vi "test-SwerveDrvPoseEst2-Test2.vi"(8 "error in (no error)":errorcluster) -> (0 "error out":errorcluster, 3 "Test Passed":bool)   [LabVIEW 2019]
uses:
  <vilib>/Rock Robotics/WPI/ThirdParty/JAS_Junk/TrajLib/Trajectory_Library.lvlib
panel:
  out "max x error":dbl
  out "max y err":dbl
  out "Y Error":dbl[](array[numeric])
  out "X error":dbl[](array[numeric])
  out "Total":i32
  out "Total passed":i32
  out "Sub error":bool
  out "End Y pos passed":bool
  out "End X pos passed":bool
  out "AddVisionCount":i32
  out "TotalTImeSecs 2":dbl
  out "BenchProcessing \nTimer Per Pass":dbl
  out "BenchTotalTime":dbl
  out "BenchTotalPasses":dbl
  out "MaxErrPassed":bool
  out "MeanPassed":bool
  out "ErrorSumNormalized":dbl
  out "Error Sum":dbl
  out "Max Error":dbl
  out "VIsionMeasCount":i32
  out "TotalTImeSecs":dbl
  out "Position Graph":cluster{dbl[], dbl[]}[](graph)
  out "PoseEst2NewErr":errorcluster
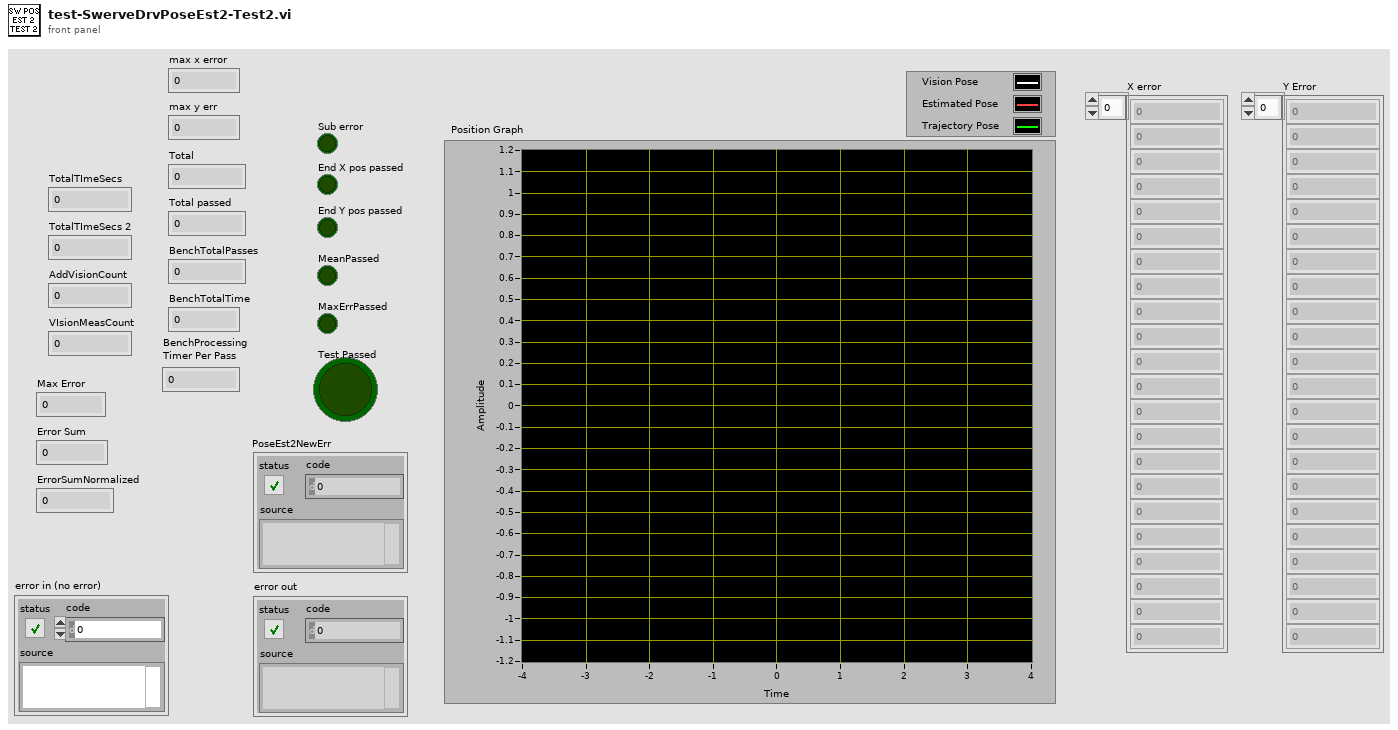
[diagram p1: front panel]
types:
  T1 = typedef "Trajectory_Library.lvlib/TRANSLATION2D.ctl" = cluster{"X":dbl, "Y":dbl}
  T2 = typedef "Trajectory_Library.lvlib/ROTATION2D.ctl" = cluster{"VALUE":dbl, "COS":dbl, "SIN":dbl}
  T3 = typedef "Trajectory_Library.lvlib/SWERVE_DRIVE_MODULE_POSITION.ctl" = cluster{"Distance":dbl, "Angle":T2, "P":bool}
  T4 = typedef "Trajectory_Library.lvlib/SWERVE_DRIVE_KINEMATICS.ctl" = cluster{"NumModules":i32, "InverseKinematics":T5, "ForwardKinematics":T5, "Modules":T1[], "PrevCoR":T1, "SavedModuleStates":T6[]}
  T5 = typedef "NI_Matrix.lvlib/RealMatrix.ctl" = dbl[][]
  T6 = typedef "Trajectory_Library.lvlib/SWERVE_DRIVE_MODULE_STATE.ctl" = cluster{"Speed":dbl, "Angle":T2}
  T7 = typedef "Trajectory_Library.lvlib/POSE2D.ctl" = cluster{"TRANSLATION":T1, "ROTATION":T2}
  T8 = typedef "Trajectory_Library.lvlib/TRAJ_CONFIG.ctl" = cluster{"MaxVelocity":dbl, "Max Acceleration":dbl, "StartVelocity":dbl, "End Velocity":dbl, "Reversed":bool, "Constraints":variant[]}
  T9 = typedef "Trajectory_Library.lvlib/SWERVE_DRIVE_POSE_EST2.ctl" = cluster{"M_Vision_K":T5, "m_nominal_dT":dbl, "m_PrevTime_Sec":dbl, "Pose_Buffer":T10, "Swerve_Drive_Kinematics":T4, "Swerve_Drive_Odom":T11, "M_Q":T5, "NumModules":i32}
  T10 = typedef "Trajectory_Library.lvlib/TIME_INTERPOLATABLE_VARIANT.ctl" = cluster{"TimeStamps":dbl[], "DataArray":variant[], "Min_TimeStamp":dbl, "Max_TimeStamp":dbl, "ItemCount":i32, "MaxBufferTime":dbl}
  T11 = typedef "Trajectory_Library.lvlib/SWERVE_DRIVE_ODOMETRY.ctl" = cluster{"POSE":T7, "GyroOffset":T2, "PreviousAngle":T2, "PrevModulePositions":T3[], "NumModules":i32}
  T12 = typedef "Trajectory_Library.lvlib/TRAJECTORY.ctl" = cluster{"TotalTImeSecs":dbl, "States":T13[]}
  T13 = typedef "Trajectory_Library.lvlib/TRAJ_STATE.ctl" = cluster{"TimeSeconds":dbl, "Velocity":dbl, "Acceleration":dbl, "POSE":T7, "Curvature":dbl}
  T14 = typedef "Trajectory_Library.lvlib/TRANSFORM2D.ctl" = cluster{"TRANSLATION":T1, "ROTATION":T2, "xF":bool}
  T15 = cluster{"MaxErrPassed":bool, "MeanPassed":bool, "Error Sum":dbl, "ErrorSumNormalized":dbl, "Max Error":dbl, "AddVisionCount":i32, "VIsionApplyCount":i32, "BenchTotalPasses":dbl, "BenchTotalTime":dbl, "BenchProcessing \nTimer Per Pass":dbl, "TotalTImeSecs":dbl, "End X pos passed":bool, "End Y pos passed":bool, "Sub error":bool, "End X Dev":dbl, "End Y Dev":dbl}
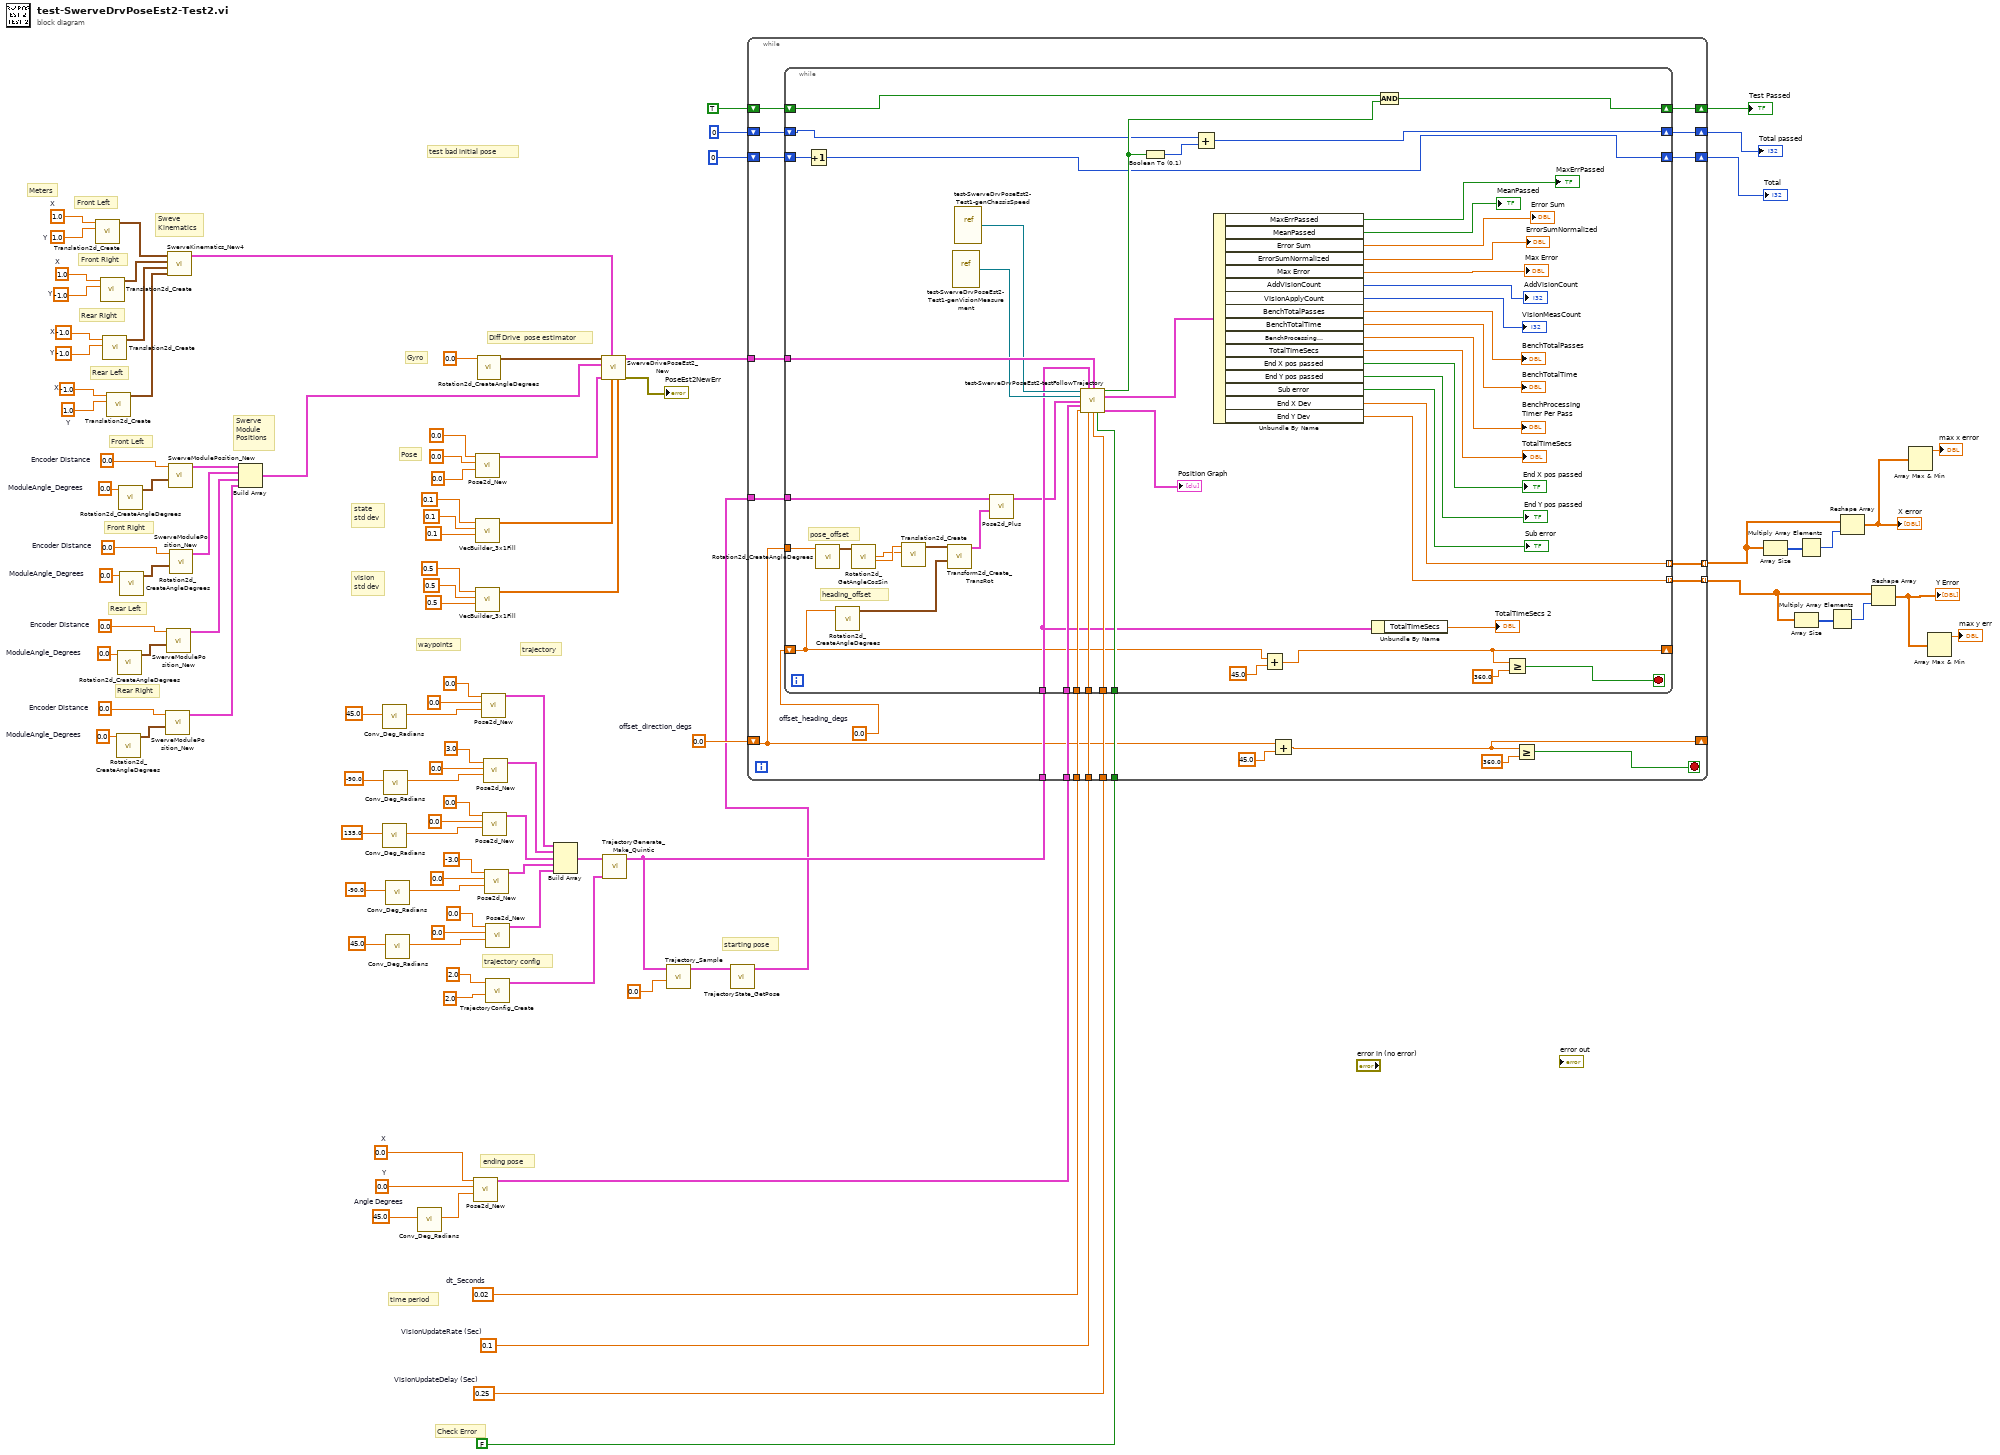
[diagram p0: block diagram]
diagram:
  w10 = -1.0  # X
  w9 = 1.0  # Y
  w8 = -1.0  # X
  w7 = -1.0  # Y
  w6 = 1.0  # X
  w5 = -1.0  # Y
  w4 = 1.0  # X
  w3 = 1.0  # Y
  w27 = 0.0  # ModuleAngle_Degrees
  w25 = 0.0  # Encoder Distance
  w24 = 0.0  # ModuleAngle_Degrees
  w22 = 0.0  # Encoder Distance
  w21 = 0.0  # ModuleAngle_Degrees
  w19 = 0.0  # Encoder Distance
  w17 = 0.0  # ModuleAngle_Degrees
  w15 = 0.0  # Encoder Distance
  w48 = 0.0  # offset_direction_degs
  w53 = 0.25  # VisionUpdateDelay (Sec)
  w54 = 0.1  # VisionUpdateRate (Sec)
  w59 = 0.0  # X
  w58 = 0.0  # Y
  w56 = 45.0  # Angle Degrees
  w60 = 0.02  # dt_Seconds
  # "Meters"
  # "Sweve\nKinematics"
  # "Rear Right"
  # "Rear Left"
  # "Front Right"
  # "Front Left"
  # "Front Left"
  # "Swerve\nModule\nPositions"
  # "Rear Right"
  # "Rear Left"
  # "Front Right"
  # "test bad initial pose"
  # "starting pose"
  # "Check Error"
  # "ending pose"
  # "state \nstd dev"
  # "time period"
  # "vision \nstd dev"
  # "Pose"
  # "Gyro"
  # "Diff Drive  pose estimator"
  # "trajectory config"
  # "trajectory"
  # "waypoints"
  n1 = call <vilib>:"Translation2d_Create.vi"("Y"=w3, "X"=w4) -> ("TRANSLATION"=w11:T1)  [unwired: 9 in]
  n2 = call <vilib>:"Translation2d_Create.vi"("Y"=w5, "X"=w6) -> ("TRANSLATION"=w12:T1)  [unwired: 9 in]
  n3 = call <vilib>:"Translation2d_Create.vi"("Y"=w7, "X"=w8) -> ("TRANSLATION"=w13:T1)  [unwired: 9 in]
  n4 = call <vilib>:"Translation2d_Create.vi"("Y"=w9, "X"=w10) -> ("TRANSLATION"=w14:T1)  [unwired: 9 in]
  n5 = call <vilib>:"Rotation2d_CreateAngleDegrees.vi"("Angle_Degrees"=w27) -> ("ROTATION"=w26:T2)  [unwired: 10 in]
  n6 = call <vilib>:"Rotation2d_CreateAngleDegrees.vi"("Angle_Degrees"=w24) -> ("ROTATION"=w23:T2)  [unwired: 10 in]
  n7 = call <vilib>:"Rotation2d_CreateAngleDegrees.vi"("Angle_Degrees"=w17) -> ("ROTATION"=w16:T2)  [unwired: 10 in]
  n8 = call <vilib>:"Rotation2d_CreateAngleDegrees.vi"("Angle_Degrees"=w21) -> ("ROTATION"=w20:T2)  [unwired: 10 in]
  n9 = call <vilib>:"SwerveModulePosition_New.vi"("ROTATION"=w26, "Distance"=w25) -> ("SWERVE_DRIVE_MODULE_POSITION"=w30:T3)  [unwired: 9 in]
  n10 = call <vilib>:"SwerveModulePosition_New.vi"("ROTATION"=w23, "Distance"=w22) -> ("SWERVE_DRIVE_MODULE_POSITION"=w29:T3)  [unwired: 9 in]
  n11 = call <vilib>:"SwerveKinematics_New4.vi"("wheel 3"=w14, "wheel 2"=w13, "wheel 1"=w12, "wheel 0"=w11) -> ("SWERVE_DRIVE_KINEMATICS"=w2:T4)  [unwired: 7 in]
  n12 = call <vilib>:"SwerveModulePosition_New.vi"("ROTATION"=w16, "Distance"=w15) -> ("SWERVE_DRIVE_MODULE_POSITION"=w18:T3)  [unwired: 9 in]
  n13 = call <vilib>:"SwerveModulePosition_New.vi"("ROTATION"=w20, "Distance"=w19) -> ("SWERVE_DRIVE_MODULE_POSITION"=w28:T3)  [unwired: 9 in]
  n14 = Build Array(w18, w28, w29, w30) -> (w1:T3[])
  n15 = call <vilib>:"Conv_Deg_Radians.vi"("Degress"=45.0 ("Heading")) -> ("Radians"=w82:dbl)  [unwired: 10 in]
  n16 = call <vilib>:"Conv_Deg_Radians.vi"("Degress"=135.0 ("Heading")) -> ("Radians"=w90:dbl)  [unwired: 10 in]
  n17 = call <vilib>:"Conv_Deg_Radians.vi"("Degress"=-90.0 ("Heading")) -> ("Radians"=w86:dbl)  [unwired: 10 in]
  n18 = call <vilib>:"Conv_Deg_Radians.vi"("Degress"=-90.0 ("Heading")) -> ("Radians"=w94:dbl)  [unwired: 10 in]
  n19 = call <vilib>:"Conv_Deg_Radians.vi"("Degress"=45.0 ("Heading")) -> ("Radians"=w98:dbl)  [unwired: 10 in]
  n20 = call <vilib>:"Conv_Deg_Radians.vi"("Degress"=w56) -> ("Radians"=w57:dbl)  [unwired: 10 in]
  n21 = call <vilib>:"Pose2d_New.vi"("Heading"=w57, "Y"=w58, "X"=w59) -> ("out POSe"=w55:T7)  [unwired: 8 in]
  n22 = call <vilib>:"Pose2d_New.vi"("Heading"=0.0, "Y"=0.0, "X"=0.0) -> ("out POSe"=w68:T7)  [unwired: 8 in]
  n23 = call <vilib>:"VecBuilder_3x1Fill.vi"("R2"=0.1 ("element"), "R1"=0.1 ("element"), "R0"=0.1 ("element")) -> ("output matrix"=w63:T5)  [unwired: 8 in]
  n24 = call <vilib>:"VecBuilder_3x1Fill.vi"("R2"=0.5 ("element"), "R1"=0.5 ("element"), "R0"=0.5 ("element")) -> ("output matrix"=w62:T5)  [unwired: 8 in]
  n25 = call <vilib>:"Rotation2d_CreateAngleDegrees.vi"("Angle_Degrees"=0.0) -> ("ROTATION"=w67:T2)  [unwired: 10 in]
  n26 = call <vilib>:"Pose2d_New.vi"("Heading"=w82, "Y"=0.0, "X"=0.0) -> ("out POSe"=w81:T7)  [unwired: 8 in]
  n27 = call <vilib>:"Pose2d_New.vi"("Heading"=w90, "Y"=0.0, "X"=0.0) -> ("out POSe"=w78:T7)  [unwired: 8 in]
  n28 = call <vilib>:"Pose2d_New.vi"("Heading"=w86, "Y"=0.0, "X"=3.0) -> ("out POSe"=w79:T7)  [unwired: 8 in]
  n29 = call <vilib>:"Pose2d_New.vi"("Heading"=w94, "Y"=0.0, "X"=-3.0) -> ("out POSe"=w77:T7)  [unwired: 8 in]
  n30 = call <vilib>:"Pose2d_New.vi"("Heading"=w98, "Y"=0.0, "X"=0.0) -> ("out POSe"=w103:T7)  [unwired: 8 in]
  n31 = call <vilib>:"TrajectoryConfig_Create.vi"("MaxAcceleration"=2.0, "MaxVelocity"=2.0) -> ("TRAJECTORY_CONFIG"=w100:T8)  [unwired: 9 in]
  n32 = Build Array(w81, w79, w78, w77, w103) -> (w101:T7[])
  n33 = call <vilib>:"SwerveDrivePoseEst2_New.vi"("VisionMeasurementStdDevs"=w62, "StateStdDevs"=w63, "SWERVE_DRIVE_KINEMATICS"=w2, "InitialPose"=w68, "Module Positions"=w1, "gyroAngle"=w67) -> ("Error"=→"PoseEst2NewErr":errorcluster, "SwerveDrivePoseEstimate"=w61:T9)  [unwired: 4 in]
  n34 = call <vilib>:"TrajectoryGenerate_Make_Quintic.vi"("traj_config"=w100, "waypointPOSE"=w101) -> ("TRAJECTORY"=w51:T12)  [unwired: 8 in, 1 out]
  n35 = call <vilib>:"Trajectory_Sample.vi"("Time"=0.0, "InputTRAJECTORY"=w51) -> ("OutputTRAJ_STATE"=w49:T13)  [unwired: 9 in]
  n36 = call <vilib>:"TrajectoryState_GetPose.vi"("TRAJ_STATE"=w49) -> ("TrajStatePose"=w47:T7)  [unwired: 10 in]
  n37 = while {
    tunnel: w61 -> [w127]
    tunnel: w60 -> [w126]
    tunnel: w55 -> [w125]
    tunnel: w54 -> [w124]
    tunnel: w53 -> [w123]
    tunnel: FALSE -> [w122]
    tunnel: w51 -> [w121]
    shift-right: [w116] -> _
    shift-left: w48 -> [w114]
    tunnel: w47 -> [w115]
    shift-right: [w112] -> w45
    shift-left: TRUE -> [w113]
    shift-right: [w110] -> w43
    shift-left: 0 -> [w111]
    shift-right: [w108] -> w41
    shift-left: 0 -> [w109]
    tunnel: [w107] -> w39 mode=indexing
    tunnel: [w106] -> w35 mode=indexing
    stop <- w118 stop-if-true
    w117 = 0.0  # offset_heading_degs
    n38 = while {
      tunnel: w127 -> [w177]
      tunnel: w126 -> [w176]
      tunnel: w125 -> [w175]
      tunnel: w124 -> [w174]
      tunnel: w123 -> [w173]
      tunnel: w122 -> [w171]
      tunnel: w121 -> [w153]
      shift-right: [w148] -> _
      shift-left: w117 -> [w146]
      tunnel: w115 -> [w139]
      tunnel: w114 -> [w144]
      shift-right: [w136] -> w112
      shift-left: w113 -> [w137]
      shift-right: [w132] -> w110
      shift-left: w111 -> [w134]
      shift-right: [w130] -> w108
      shift-left: w109 -> [w131]
      tunnel: [w129] -> w107 mode=indexing
      tunnel: [w128] -> w106 mode=indexing
      stop <- w149 stop-if-true
      # "heading_offset"
      # "pose_offset"
      n39 = Increment(x=w131) -> (x+1=w130:i32)
      n40 = call <vilib>:"Rotation2d_CreateAngleDegrees.vi"("Angle_Degrees"=w144) -> ("ROTATION"=w145:T2)  [unwired: 10 in]
      n41 = call <vilib>:"Rotation2d_CreateAngleDegrees.vi"("Angle_Degrees"=w146) -> ("ROTATION"=w141:T2)  [unwired: 10 in]
      n42 = call <vilib>:"Rotation2d_GetAngleCosSin.vi"("in ROTATION"=w145) -> ("Cosine"=w143:dbl, "Sine"=w142:dbl)  [unwired: 8 in, 1 out]
      n43 = call <vilib>:"Translation2d_Create.vi"("Y"=w142, "X"=w143) -> ("TRANSLATION"=w147:T1)  [unwired: 9 in]
      n44 = call <vilib>:"Transform2d_Create_TransRot.vi"("ROTATION"=w141, "TRANSLATION"=w147) -> ("TRANSFORM"=w140:T14)  [unwired: 9 in]
      n45 = vi-ref "test-SwerveDrvPoseEst2-Test1-genVisionMeasurement.vi"() -> (w169:refnum<vi>)
      n46 = vi-ref "test-SwerveDrvPoseEst2-Test1-genChassisSpeed.vi"() -> (w170:refnum<vi>)
      n47 = call <vilib>:"Pose2d_Plus.vi"("other TRANSFORM"=w140, "in POSE"=w139) -> ("out POSE"=w138:T7)  [unwired: 9 in]
      n48 = call "test-SwerveDrvPoseEst2-testFollowTrajectory.vi"("chassisSpeedsGenerator"=w170, "TRAJECTORY"=w153, "SwerveDrivePoseEstimate2"=w177, "genVisionMeasurement"=w169, "StartingPose"=w138, "EndingPose"=w175, "dt_Seconds"=w176, "VisionUpdateRate"=w174, "VisionUpdateDelay"=w173, "CheckError"=w171) -> ("Test Passed"=w135:bool, "Output Data"=w167:T15, "DataForGraph"=→"Position Graph":cluster{dbl[], dbl[]}[])  [unwired: 3 in]
      n49 = Boolean To (0,1)(Boolean=w135) -> (0, 1=w133:i16)
      n50 = Add(x=w134, y=w133) -> (x+y=w132:i32)
      n51 = Unbundle By Name(w167) -> ("MaxErrPassed"=→"MaxErrPassed":bool, "MeanPassed"=→"MeanPassed":bool, "Error Sum"=→"Error Sum":dbl, "ErrorSumNormalized"=→"ErrorSumNormalized":dbl, "Max Error"=→"Max Error":dbl, "AddVisionCount"=→"AddVisionCount":i32, "VIsionApplyCount"=→"VIsionMeasCount":i32, "BenchTotalPasses"=→"BenchTotalPasses":dbl, "BenchTotalTime"=→"BenchTotalTime":dbl, "BenchProcessing \nTimer Per Pass"=→"BenchProcessing \nTimer Per Pass":dbl, "TotalTImeSecs"=→"TotalTImeSecs":dbl, "End X pos passed"=→"End X pos passed":bool, "End Y pos passed"=→"End Y pos passed":bool, "Sub error"=→"Sub error":bool, "End X Dev"=w129:dbl, "End Y Dev"=w128:dbl)
      n52 = Add(x=w146, y=45.0) -> (x+y=w148:dbl)
      n53 = Unbundle By Name(w153) -> ("TotalTImeSecs"=→"TotalTImeSecs 2":dbl)
      n54 = And(x=w137, y=w135) -> (x .and. y?=w136:bool)
      n55 = Greater Or Equal?(x=w148, y=360.0) -> (x >= y?=w149:bool)
    }
    n56 = Add(x=w114, y=45.0) -> (x+y=w116:dbl)
    n57 = Greater Or Equal?(x=w116, y=360.0) -> (x >= y?=w118:bool)
  }
  "Test Passed" <- w45
  "Total passed" <- w43
  "Total" <- w41
  n58 = Array Size(array=w39) -> (size(s)=w40:i32[])
  n59 = Array Size(array=w35) -> (size(s)=w37:i32[])
  n60 = Multiply Array Elements(1:w40) -> (0:w38:i32)
  n61 = Multiply Array Elements(1:w37) -> (0:w36:i32)
  n62 = Reshape Array(w39, w38) -> (w34:dbl[])
  "X error" <- w34
  n63 = Reshape Array(w35, w36) -> (w33:dbl[])
  "Y Error" <- w33
  n64 = Array Max & Min(array=w34) -> (max value=→"max x error":dbl)  [unwired: 3 out]
  n65 = Array Max & Min(array=w33) -> (max value=→"max y err":dbl)  [unwired: 3 out]
